vi "map_diag.vi"() -> ()   [LabVIEW 2015]
panel:
  in  "Panello o pcb?":bool
  in  "y inizio":bool
  in  "Positioning Done":bool
  in  "x inizio":bool
  in  "y inizio":bool
  in  "Positioning Done":bool
  in  "y inizio":bool
  in  "Positioning Done":bool
  in  "KILL":bool
  in  "PAUSE":bool
  in  "RESUME":bool
  in  "QUIT":bool
  in  "Positioning Done":bool
  in  "z inizio":bool
  in  "y inizio":bool
  in  "x inizio":bool
  in  "End":bool
  in  "zero z - end":bool
  in  "zero x - end":bool
  in  "zero y - end":bool
  out "output":string
  out "command":string
  in  "zero done":bool
  in  "zero z":bool
  in  "zero x":bool
  in  "zero y":bool
  # "In alto: TRUE ---> Panello"
  # "In basso: FALSE ---> PCB"
  # "Comandi di emergenza"
  # "Posiziono in zero"
  # "Vado al punto di partenza\nDiagonale Left Internal"
  # "Vado al punto di partenza\nDiagonale Right Internal"
  # "Vado al punto di partenza\nDiagonale Left External"
  # "Vado al punto di partenza\nDiagonale Right External"
  # "Ritorno a zero"
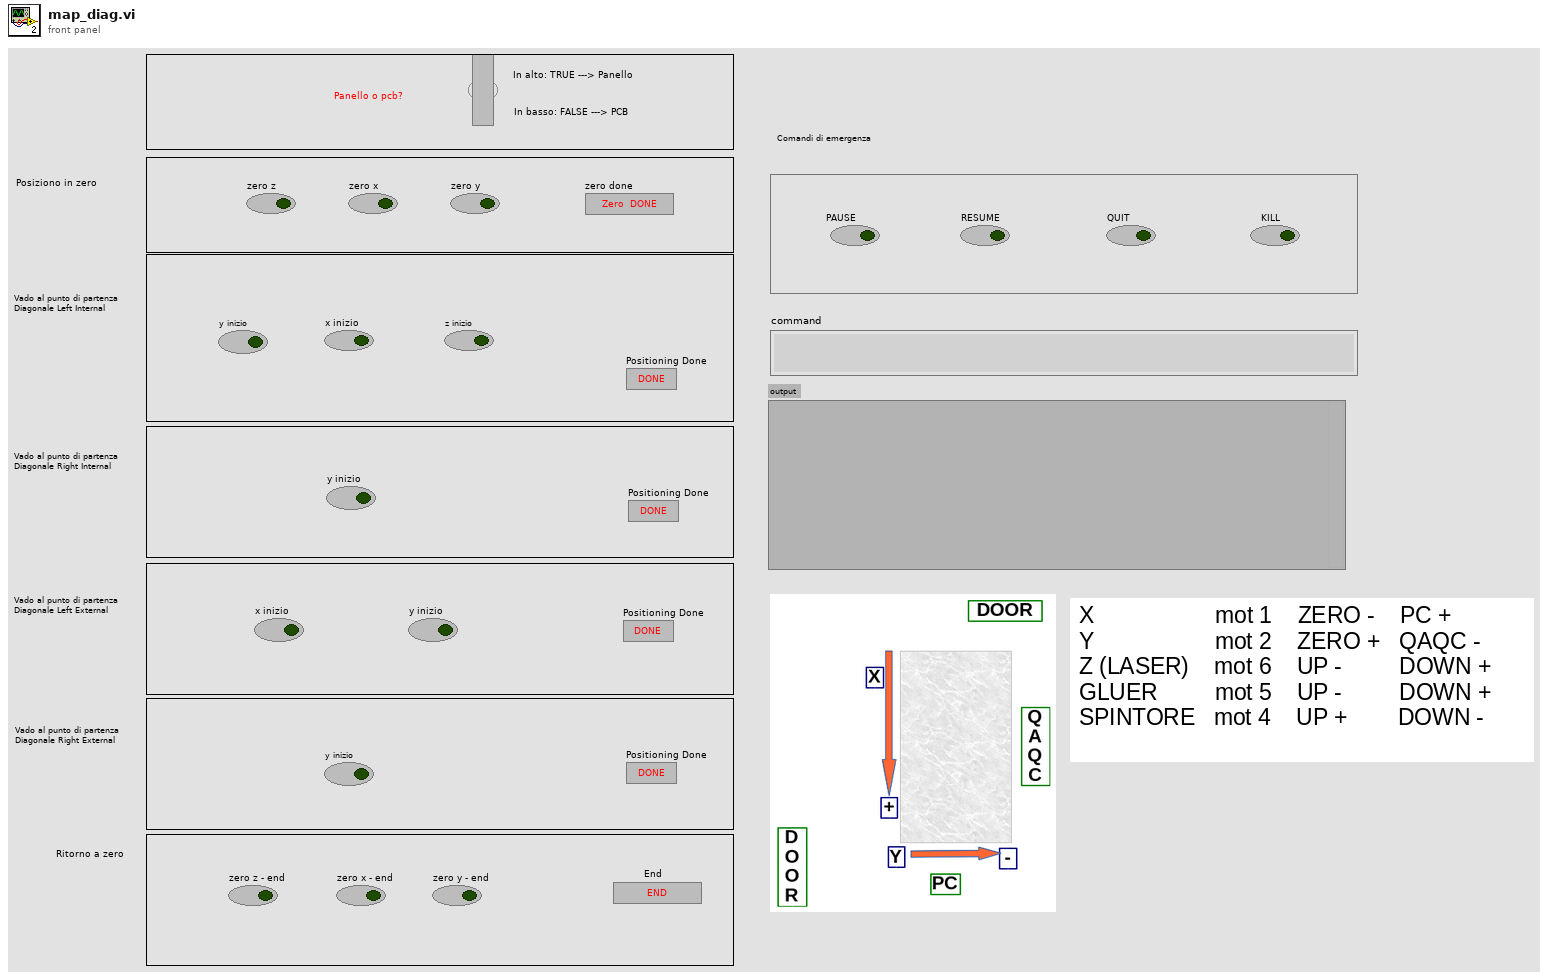
[diagram p1: front panel]
types:
  T1 = enum16{"open", "replace", "create", "open or create", "replace or create", "replace or create with confirmation"}
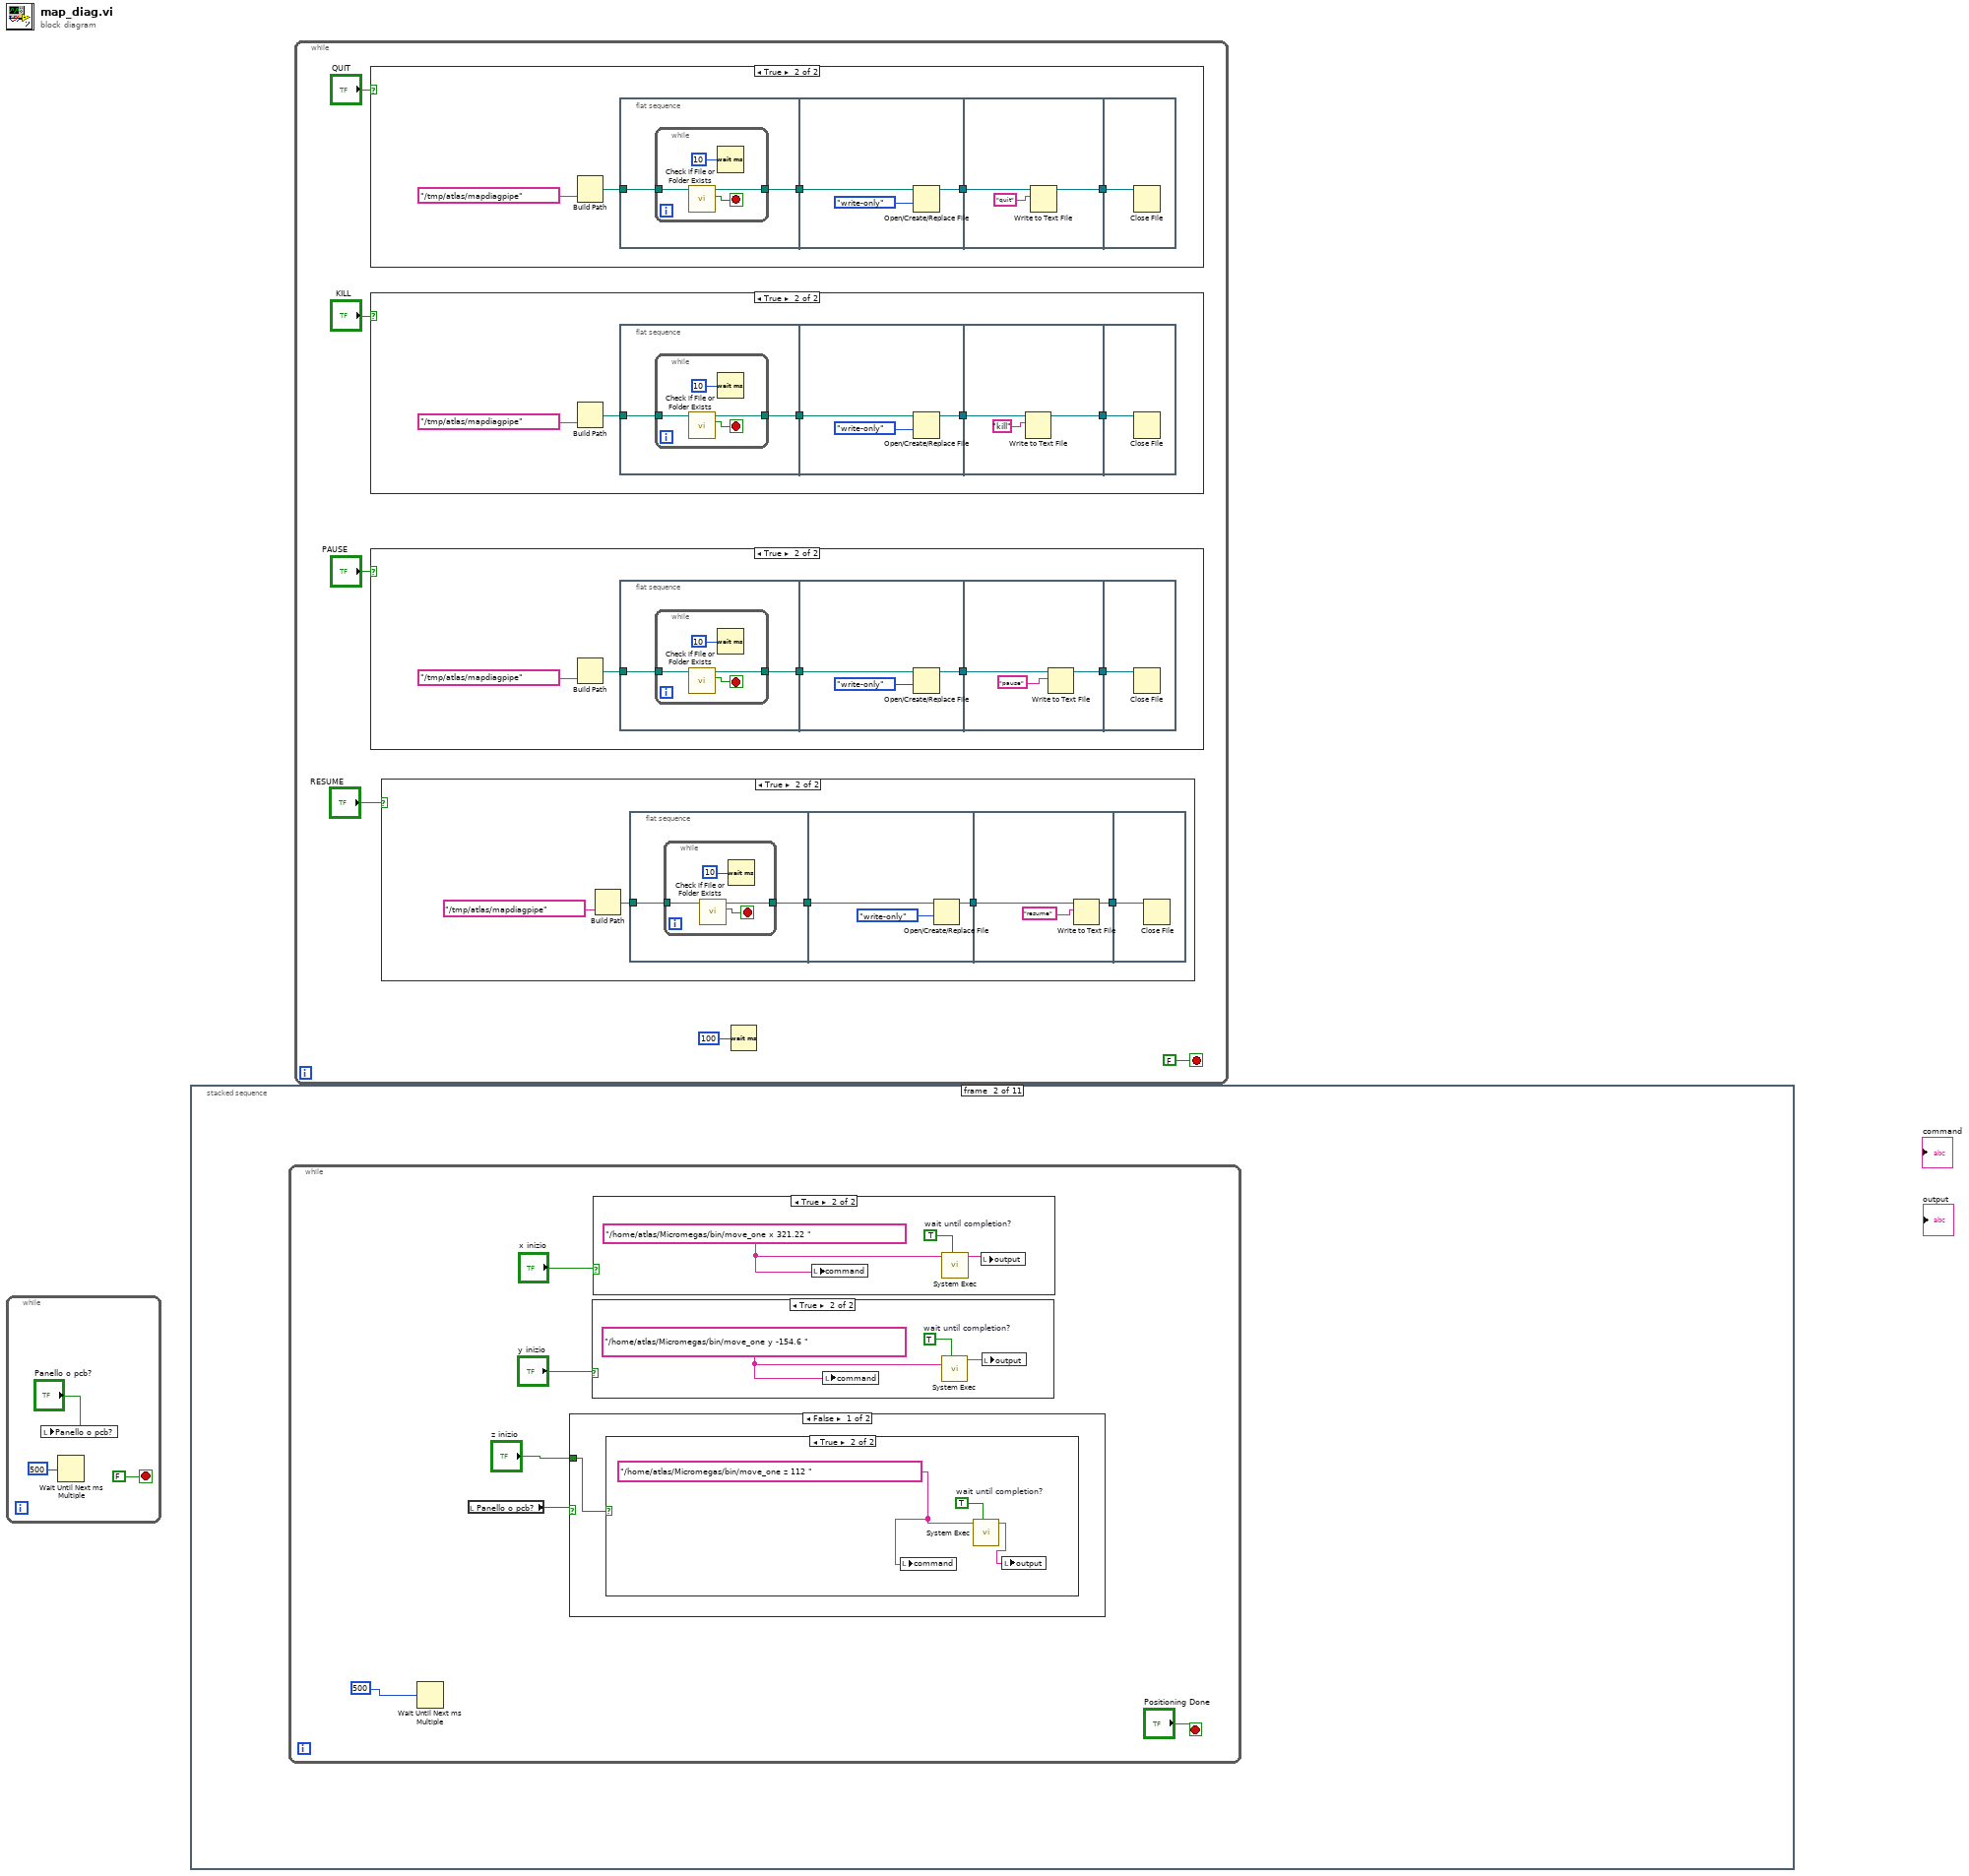
[diagram p0: block diagram]
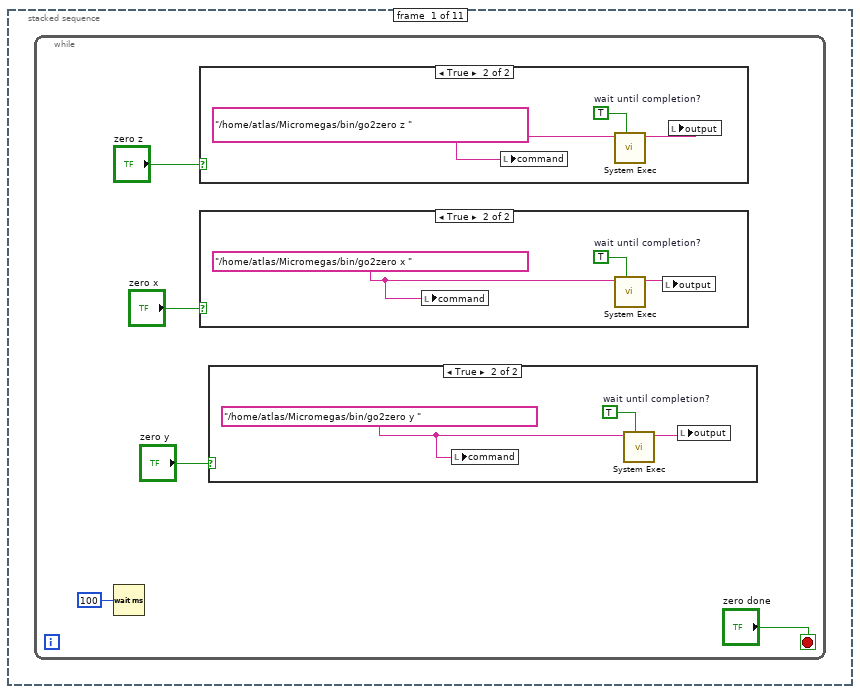
[diagram p6: hidden frame]
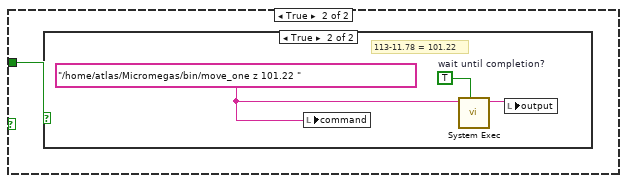
[diagram p11: hidden frame]
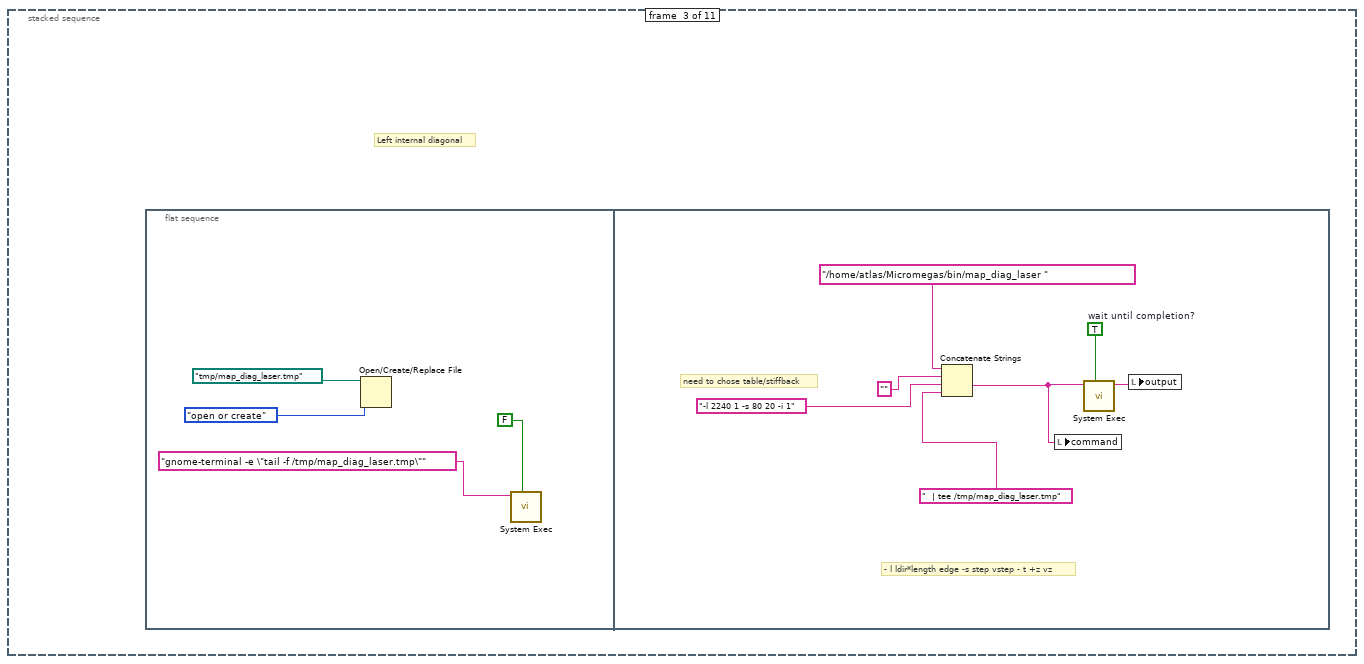
[diagram p15: hidden frame]
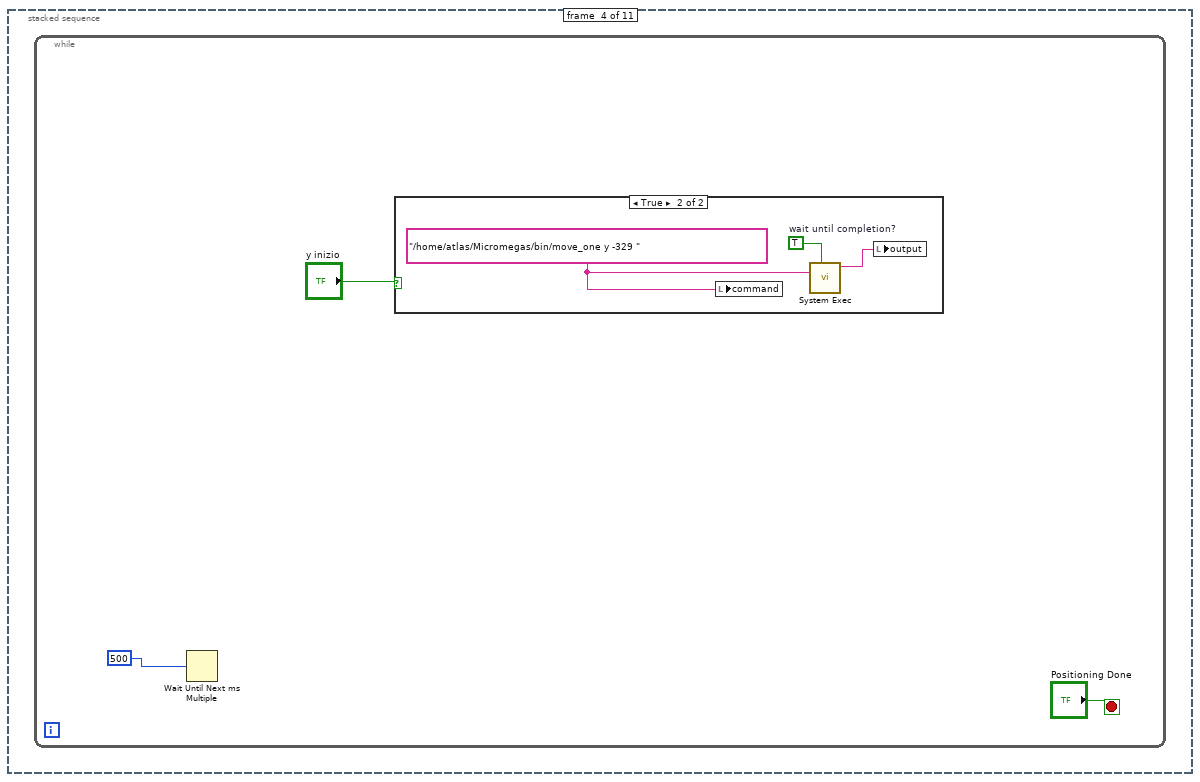
[diagram p16: hidden frame]
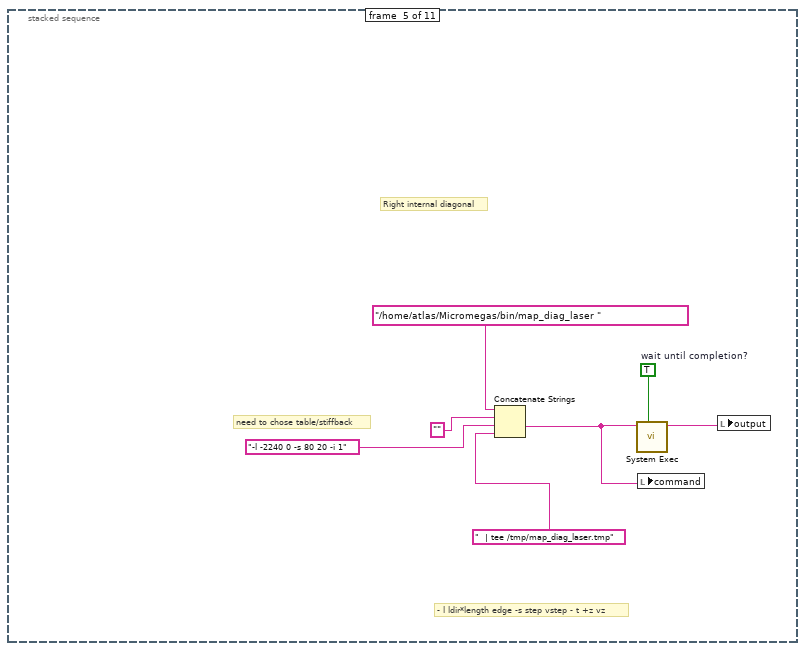
[diagram p18: hidden frame]
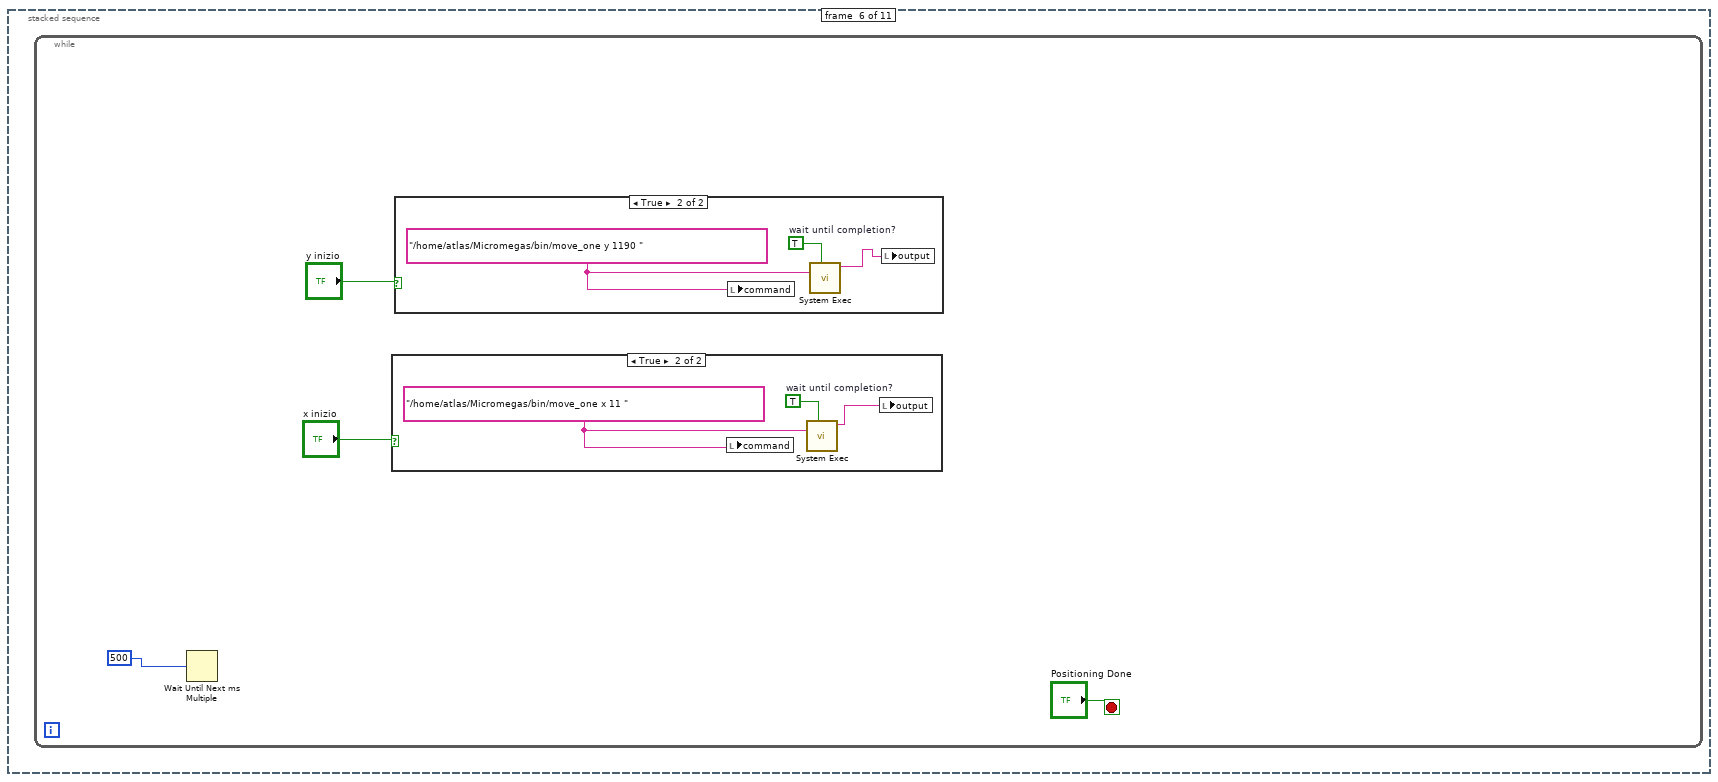
[diagram p19: hidden frame]
diagram:
  n1 = while {
    stop <- FALSE stop-if-true
    n2 = local write "Panello o pcb?"("Panello o pcb?") -> ()
    n3 = Wait Until Next ms Multiple(millisecond multiple=u32 500) -> ()  [unwired: 1 out]
  }
  n4 = stacked-sequence {
    frame #0 {
      n5 = while {
        stop <- "zero done" stop-if-true
        n6 = Wait (ms)(milliseconds to wait=u32 100) -> ()  [unwired: 1 out]
        n7 = case shown="True" "zero z" {
          frame False {
          }
          frame True {
            w16 = "/home/atlas/Micromegas/bin/go2zero z " ("string")
            w17 = TRUE  # wait until completion?
            n8 = local write "command"(w16) -> ()
            n9 = call <vilib>:"System Exec.vi"("wait until completion? (T)"=w17, "command line"=w16) -> ("standard output"=w15:string)  [unwired: 6 in, 3 out]
            n10 = local write "output"(w15) -> ()
          }
        }
        n11 = case shown="True" "zero x" {
          frame False {
          }
          frame True {
            w13 = "/home/atlas/Micromegas/bin/go2zero x " ("string")
            w14 = TRUE  # wait until completion?
            n12 = local write "command"(w13) -> ()
            n13 = call <vilib>:"System Exec.vi"("wait until completion? (T)"=w14, "command line"=w13) -> ("standard output"=w12:string)  [unwired: 6 in, 3 out]
            n14 = local write "output"(w12) -> ()
          }
        }
        n15 = case shown="True" "zero y" {
          frame False {
          }
          frame True {
            w10 = "/home/atlas/Micromegas/bin/go2zero y " ("string")
            w11 = TRUE  # wait until completion?
            n16 = local write "command"(w10) -> ()
            n17 = call <vilib>:"System Exec.vi"("wait until completion? (T)"=w11, "command line"=w10) -> ("standard output"=w9:string)  [unwired: 6 in, 3 out]
            n18 = local write "output"(w9) -> ()
          }
        }
      }
    }
    frame #1 {
      n19 = while {
        stop <- "Positioning Done" stop-if-true
        n20 = Wait Until Next ms Multiple(millisecond multiple=u32 500 ("millisecond timer value")) -> ()  [unwired: 1 out]
        n21 = local read "Panello o pcb?"() -> (w18:bool)
        n22 = case shown="False" w18 {
          tunnel: "z inizio" -> [w24 w28]
          frame False {
            n23 = case shown="True" w24 {
              frame False {
              }
              frame True {
                w27 = TRUE  # wait until completion?
                w25 = "/home/atlas/Micromegas/bin/move_one z 112 " ("string")
                n24 = local write "command"(w25) -> ()
                n25 = call <vilib>:"System Exec.vi"("wait until completion? (T)"=w27, "command line"=w25) -> ("standard output"=w26:string)  [unwired: 6 in, 3 out]
                n26 = local write "output"(w26) -> ()
              }
            }
          }
          frame True {
            n27 = case shown="True" w28 {
              frame False {
              }
              frame True {
                w29 = "/home/atlas/Micromegas/bin/move_one z 101.22 " ("string")
                w31 = TRUE  # wait until completion?
                # "113-11.78 = 101.22"
                n28 = local write "command"(w29) -> ()
                n29 = call <vilib>:"System Exec.vi"("wait until completion? (T)"=w31, "command line"=w29) -> ("standard output"=w30:string)  [unwired: 6 in, 3 out]
                n30 = local write "output"(w30) -> ()
              }
            }
          }
        }
        n31 = case shown="True" "y inizio" {
          frame False {
          }
          frame True {
            w32 = "/home/atlas/Micromegas/bin/move_one y -154.6 " ("string")
            w34 = TRUE  # wait until completion?
            n32 = local write "command"(w32) -> ()
            n33 = call <vilib>:"System Exec.vi"("wait until completion? (T)"=w34, "command line"=w32) -> ("standard output"=w33:string)  [unwired: 6 in, 3 out]
            n34 = local write "output"(w33) -> ()
          }
        }
        n35 = case shown="True" "x inizio" {
          frame False {
          }
          frame True {
            w35 = "/home/atlas/Micromegas/bin/move_one x 321.22 " ("string")
            w37 = TRUE  # wait until completion?
            n36 = local write "command"(w35) -> ()
            n37 = call <vilib>:"System Exec.vi"("wait until completion? (T)"=w37, "command line"=w35) -> ("standard output"=w36:string)  [unwired: 6 in, 3 out]
            n38 = local write "output"(w36) -> ()
          }
        }
      }
    }
    frame #2 {
      # "Left internal diagonal"
      n39 = flat-sequence {
        frame #0 {
          n40 = Open/Create/Replace File(file path (use dialog)=path "/tmp/map_diag_laser.tmp", operation (0:open)=T1."open or create") -> ()  [unwired: 4 in, 3 out]
          n41 = call <vilib>:"System Exec.vi"("wait until completion? (T)"=FALSE, "command line"="gnome-terminal -e \"tail -f /tmp/map_diag_laser.tmp\"") -> ()  [unwired: 6 in, 4 out]
        }
        frame #1 {
          w48 = TRUE  # wait until completion?
          # "need to chose table/stiffback"
          # "- l ldir*length edge -s step vstep - t +z vz"
          n42 = Concatenate Strings("/home/atlas/Micromegas/bin/map_diag_laser " ("string"), "" ("string"), "-l 2240 1 -s 80 20 -i 1" ("string"), "  | tee /tmp/map_diag_laser.tmp" ("string")) -> (w45:string)
          n43 = local write "command"(w45) -> ()
          n44 = call <vilib>:"System Exec.vi"("wait until completion? (T)"=w48, "command line"=w45) -> ("standard output"=w46:string)  [unwired: 6 in, 3 out]
          n45 = local write "output"(w46) -> ()
        }
      }
    }
    frame #3 {
      n46 = while {
        stop <- "Positioning Done" stop-if-true
        n47 = Wait Until Next ms Multiple(millisecond multiple=u32 500 ("millisecond timer value")) -> ()  [unwired: 1 out]
        n48 = case shown="True" "y inizio" {
          frame False {
          }
          frame True {
            w52 = "/home/atlas/Micromegas/bin/move_one y -329 " ("string")
            w54 = TRUE  # wait until completion?
            n49 = local write "command"(w52) -> ()
            n50 = call <vilib>:"System Exec.vi"("wait until completion? (T)"=w54, "command line"=w52) -> ("standard output"=w53:string)  [unwired: 6 in, 3 out]
            n51 = local write "output"(w53) -> ()
          }
        }
      }
    }
    frame #4 {
      w61 = TRUE  # wait until completion?
      # "Right internal diagonal"
      # "need to chose table/stiffback"
      # "- l ldir*length edge -s step vstep - t +z vz"
      n52 = Concatenate Strings("/home/atlas/Micromegas/bin/map_diag_laser " ("string"), "" ("string"), "-l -2240 0 -s 80 20 -i 1" ("string"), "  | tee /tmp/map_diag_laser.tmp" ("string")) -> (w55:string)
      n53 = call <vilib>:"System Exec.vi"("wait until completion? (T)"=w61, "command line"=w55) -> ("standard output"=w56:string)  [unwired: 6 in, 3 out]
      n54 = local write "command"(w55) -> ()
      n55 = local write "output"(w56) -> ()
    }
    frame #5 {
      n56 = while {
        stop <- "Positioning Done" stop-if-true
        n57 = Wait Until Next ms Multiple(millisecond multiple=u32 500 ("millisecond timer value")) -> ()  [unwired: 1 out]
        n58 = case shown="True" "x inizio" {
          frame False {
          }
          frame True {
            w66 = "/home/atlas/Micromegas/bin/move_one x 11 " ("string")
            w68 = TRUE  # wait until completion?
            n59 = local write "command"(w66) -> ()
            n60 = call <vilib>:"System Exec.vi"("wait until completion? (T)"=w68, "command line"=w66) -> ("standard output"=w67:string)  [unwired: 6 in, 3 out]
            n61 = local write "output"(w67) -> ()
          }
        }
        n62 = case shown="True" "y inizio" {
          frame False {
          }
          frame True {
            w69 = "/home/atlas/Micromegas/bin/move_one y 1190 " ("string")
            w71 = TRUE  # wait until completion?
            n63 = local write "command"(w69) -> ()
            n64 = call <vilib>:"System Exec.vi"("wait until completion? (T)"=w71, "command line"=w69) -> ("standard output"=w70:string)  [unwired: 6 in, 3 out]
            n65 = local write "output"(w70) -> ()
          }
        }
      }
    }
    frame #6 {
      w78 = TRUE  # wait until completion?
      # "Left external diagonal"
      # "need to chose table/stiffback"
      # "- l ldir*length edge -s step vstep - t +z vz"
      n66 = Concatenate Strings("/home/atlas/Micromegas/bin/map_diag_laser " ("string"), "" ("string"), "-l 2200 1 -s 110 20 -i 1" ("string"), "  | tee /tmp/map_diag_laser.tmp" ("string")) -> (w72:string)
      n67 = call <vilib>:"System Exec.vi"("wait until completion? (T)"=w78, "command line"=w72) -> ("standard output"=w73:string)  [unwired: 6 in, 3 out]
      n68 = local write "command"(w72) -> ()
      n69 = local write "output"(w73) -> ()
    }
    frame #7 {
      n70 = while {
        stop <- "Positioning Done" stop-if-true
        n71 = Wait Until Next ms Multiple(millisecond multiple=u32 500 ("millisecond timer value")) -> ()  [unwired: 1 out]
        n72 = case shown="True" "y inizio" {
          frame False {
          }
          frame True {
            w82 = "/home/atlas/Micromegas/bin/move_one y -505 " ("string")
            w84 = TRUE  # wait until completion?
            n73 = local write "command"(w82) -> ()
            n74 = call <vilib>:"System Exec.vi"("wait until completion? (T)"=w84, "command line"=w82) -> ("standard output"=w83:string)  [unwired: 6 in, 3 out]
            n75 = local write "output"(w83) -> ()
          }
        }
      }
    }
    frame #8 {
      w91 = TRUE  # wait until completion?
      # "Right external diagonal"
      # "need to chose table/stiffback"
      # "- l ldir*length edge -s step vstep - t +z vz"
      n76 = Concatenate Strings("/home/atlas/Micromegas/bin/map_diag_laser " ("string"), "" ("string"), "-l -2200 0 -s 110 20 -i 1" ("string"), "  | tee /tmp/map_diag_laser.tmp" ("string")) -> (w85:string)
      n77 = call <vilib>:"System Exec.vi"("wait until completion? (T)"=w91, "command line"=w85) -> ("standard output"=w86:string)  [unwired: 6 in, 3 out]
      n78 = local write "command"(w85) -> ()
      n79 = local write "output"(w86) -> ()
    }
    frame #9 {
      n80 = while {
        stop <- "End" stop-if-true
        n81 = Wait (ms)(milliseconds to wait=u32 100) -> ()  [unwired: 1 out]
        n82 = case shown="True" "zero z - end" {
          frame False {
          }
          frame True {
            w104 = "/home/atlas/Micromegas/bin/go2zero z " ("string")
            w105 = TRUE  # wait until completion?
            n83 = local write "command"(w104) -> ()
            n84 = call <vilib>:"System Exec.vi"("wait until completion? (T)"=w105, "command line"=w104) -> ("standard output"=w103:string)  [unwired: 6 in, 3 out]
            n85 = local write "output"(w103) -> ()
          }
        }
        n86 = case shown="True" "zero x - end" {
          frame False {
          }
          frame True {
            w101 = "/home/atlas/Micromegas/bin/go2zero x " ("string")
            w102 = TRUE  # wait until completion?
            n87 = local write "command"(w101) -> ()
            n88 = call <vilib>:"System Exec.vi"("wait until completion? (T)"=w102, "command line"=w101) -> ("standard output"=w100:string)  [unwired: 6 in, 3 out]
            n89 = local write "output"(w100) -> ()
          }
        }
        n90 = case shown="True" "zero y - end" {
          frame False {
          }
          frame True {
            w98 = "/home/atlas/Micromegas/bin/go2zero y " ("string")
            w99 = TRUE  # wait until completion?
            n91 = local write "command"(w98) -> ()
            n92 = call <vilib>:"System Exec.vi"("wait until completion? (T)"=w99, "command line"=w98) -> ("standard output"=w97:string)  [unwired: 6 in, 3 out]
            n93 = local write "output"(w97) -> ()
          }
        }
      }
    }
    frame #10 {
      n94 = One Button Dialog(message="Per comodita`, rinominare il file (non verra` comunque sovrascritto)") -> ()  [unwired: 1 in, 1 out]
    }
  }
  n95 = while {
    stop <- FALSE stop-if-true
    n96 = case shown="True" "QUIT" {
      frame False {
      }
      frame True {
        n97 = Build Path(name or relative path="/tmp/atlas/mapdiagpipe" ("string")) -> (appended path=w167:path)  [unwired: 1 in]
        n98 = flat-sequence {
          tunnel: [w173] -> w171
          tunnel: w167 -> [w172]
          tunnel: w171 -> [w180]
          tunnel: [w178] -> w170
          tunnel: w170 -> [w183]
          tunnel: [w182] -> w169
          tunnel: w169 -> [w184]
          frame #0 {
            n99 = while {
              tunnel: [w175] -> w173
              tunnel: w172 -> [w174]
              stop <- w176 stop-if-true
              n100 = call <vilib>:"Check if File or Folder Exists.vi"("path"=w174) -> ("file or folder exists?"=w176:bool, "dup path"=w175:path)  [unwired: 8 in, 1 out]
              n101 = Wait (ms)(milliseconds to wait=u32 10) -> ()  [unwired: 1 out]
            }
          }
          frame #1 {
            n102 = Open/Create/Replace File(file path (use dialog)=w180, access (0:read/write)=enum16{"read/write", "read-only", "write-only"}."write-only") -> (refnum out=w178:refnum<file>)  [unwired: 4 in, 2 out]
          }
          frame #2 {
            n103 = Write to Text File(file (use dialog)=w183, text="quit") -> (refnum out=w182:refnum<file>)  [unwired: 2 in, 2 out]
          }
          frame #3 {
            n104 = Close File(refnum=w184) -> ()  [unwired: 1 in, 2 out]
          }
        }
      }
    }
    n105 = case shown="True" "KILL" {
      frame False {
      }
      frame True {
        n106 = Build Path(name or relative path="/tmp/atlas/mapdiagpipe" ("string")) -> (appended path=w131:path)  [unwired: 1 in]
        n107 = flat-sequence {
          tunnel: [w137] -> w135
          tunnel: w131 -> [w136]
          tunnel: w135 -> [w144]
          tunnel: [w142] -> w134
          tunnel: w134 -> [w147]
          tunnel: [w146] -> w133
          tunnel: w133 -> [w148]
          frame #0 {
            n108 = while {
              tunnel: [w139] -> w137
              tunnel: w136 -> [w138]
              stop <- w140 stop-if-true
              n109 = call <vilib>:"Check if File or Folder Exists.vi"("path"=w138) -> ("file or folder exists?"=w140:bool, "dup path"=w139:path)  [unwired: 8 in, 1 out]
              n110 = Wait (ms)(milliseconds to wait=u32 10) -> ()  [unwired: 1 out]
            }
          }
          frame #1 {
            n111 = Open/Create/Replace File(file path (use dialog)=w144, access (0:read/write)=enum16{"read/write", "read-only", "write-only"}."write-only") -> (refnum out=w142:refnum<file>)  [unwired: 4 in, 2 out]
          }
          frame #2 {
            n112 = Write to Text File(file (use dialog)=w147, text="kill") -> (refnum out=w146:refnum<file>)  [unwired: 2 in, 2 out]
          }
          frame #3 {
            n113 = Close File(refnum=w148) -> ()  [unwired: 1 in, 2 out]
          }
        }
      }
    }
    n114 = case shown="True" "PAUSE" {
      frame False {
      }
      frame True {
        n115 = Build Path(name or relative path="/tmp/atlas/mapdiagpipe" ("string")) -> (appended path=w113:path)  [unwired: 1 in]
        n116 = flat-sequence {
          tunnel: [w119] -> w117
          tunnel: w113 -> [w118]
          tunnel: w117 -> [w126]
          tunnel: [w124] -> w116
          tunnel: w116 -> [w129]
          tunnel: [w128] -> w115
          tunnel: w115 -> [w130]
          frame #0 {
            n117 = while {
              tunnel: [w121] -> w119
              tunnel: w118 -> [w120]
              stop <- w122 stop-if-true
              n118 = call <vilib>:"Check if File or Folder Exists.vi"("path"=w120) -> ("file or folder exists?"=w122:bool, "dup path"=w121:path)  [unwired: 8 in, 1 out]
              n119 = Wait (ms)(milliseconds to wait=u32 10) -> ()  [unwired: 1 out]
            }
          }
          frame #1 {
            n120 = Open/Create/Replace File(file path (use dialog)=w126, access (0:read/write)=enum16{"read/write", "read-only", "write-only"}."write-only") -> (refnum out=w124:refnum<file>)  [unwired: 4 in, 2 out]
          }
          frame #2 {
            n121 = Write to Text File(file (use dialog)=w129, text="pause") -> (refnum out=w128:refnum<file>)  [unwired: 2 in, 2 out]
          }
          frame #3 {
            n122 = Close File(refnum=w130) -> ()  [unwired: 1 in, 2 out]
          }
        }
      }
    }
    n123 = case shown="True" "RESUME" {
      frame False {
      }
      frame True {
        n124 = Build Path(name or relative path="/tmp/atlas/mapdiagpipe" ("string")) -> (appended path=w149:path)  [unwired: 1 in]
        n125 = flat-sequence {
          tunnel: [w155] -> w153
          tunnel: w149 -> [w154]
          tunnel: w153 -> [w162]
          tunnel: [w160] -> w152
          tunnel: w152 -> [w165]
          tunnel: [w164] -> w151
          tunnel: w151 -> [w166]
          frame #0 {
            n126 = while {
              tunnel: [w157] -> w155
              tunnel: w154 -> [w156]
              stop <- w158 stop-if-true
              n127 = call <vilib>:"Check if File or Folder Exists.vi"("path"=w156) -> ("file or folder exists?"=w158:bool, "dup path"=w157:path)  [unwired: 8 in, 1 out]
              n128 = Wait (ms)(milliseconds to wait=u32 10) -> ()  [unwired: 1 out]
            }
          }
          frame #1 {
            n129 = Open/Create/Replace File(file path (use dialog)=w162, access (0:read/write)=enum16{"read/write", "read-only", "write-only"}."write-only") -> (refnum out=w160:refnum<file>)  [unwired: 4 in, 2 out]
          }
          frame #2 {
            n130 = Write to Text File(file (use dialog)=w165, text="resume") -> (refnum out=w164:refnum<file>)  [unwired: 2 in, 2 out]
          }
          frame #3 {
            n131 = Close File(refnum=w166) -> ()  [unwired: 1 in, 2 out]
          }
        }
      }
    }
    n132 = Wait (ms)(milliseconds to wait=100) -> ()  [unwired: 1 out]
  }
